vi "FYP_VI_MIDI_TestCNote.vi"(7 "deviceID":u32) -> (3 "DeviceIdOut":u32)   [LabVIEW 2013]
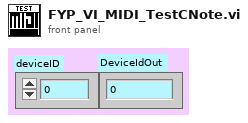
[diagram p1: front panel]
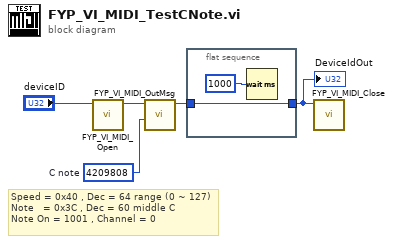
[diagram p0: block diagram]
diagram:
  w5 = 4209808  # C note
  # "Speed = 0x40 , Dec = 64 range (0 ~ 127)\nNote   = 0x3C , Dec = 60 middle C\nNote On = 1001 , Channel = 0"
  n1 = call "FYP_VI_MIDI_Open.vi"("deviceID"="deviceID") -> ("midiOut"=w3:i32)  [unwired: 5 in, 1 out]
  n2 = call "FYP_VI_MIDI_OutMsg.vi"("dwMsg dataIn"=w5, "midiOut hmo"=w3) -> ("midiOut handle"=w4:i32)  [unwired: 4 in, 1 out]
  n3 = flat-sequence {
    tunnel: w4 -> [w6]
    tunnel: [w6] -> w1
    frame #0 {
      n4 = Wait (ms)(milliseconds to wait=u32 1000) -> ()  [unwired: 1 out]
    }
  }
  n5 = call "FYP_VI_MIDI_Close.vi"("midiOut"=w1) -> ()  [unwired: 6 in, 1 out]
  "DeviceIdOut" <- w1
